vi "recipeScript versionInformation.vi"() -> (0 "verInfo":string)   [LabVIEW 2018]
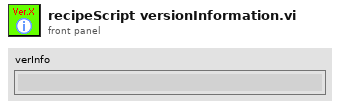
[diagram p1: front panel]
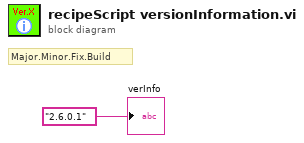
[diagram p0: block diagram]
diagram:
  # "Major.Minor.Fix.Build"
  "verInfo" <- "2.6.0.1"
